vi "Report.FileName.vi"(8 "error in (no error)":errorcluster caption="错误输入（无错误）", 11 "路径":path) -> (0 "error out":errorcluster caption="错误输出", 2 "处理文件数量":u32, 3 "ok?":bool)   [LabVIEW 2012, in "Lib_UEL.ATE.lvlib" / "Lib_Report.lvlib"]
uses:
  <vilib>/regexp/Match Regular Expression.xnode
  Lib_Report.lvlib
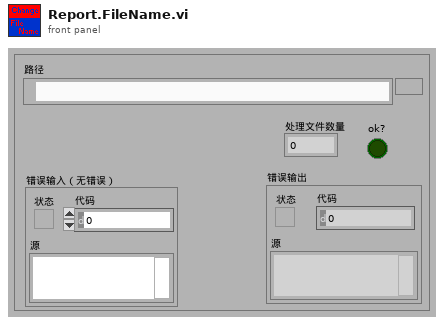
[diagram p1: front panel]
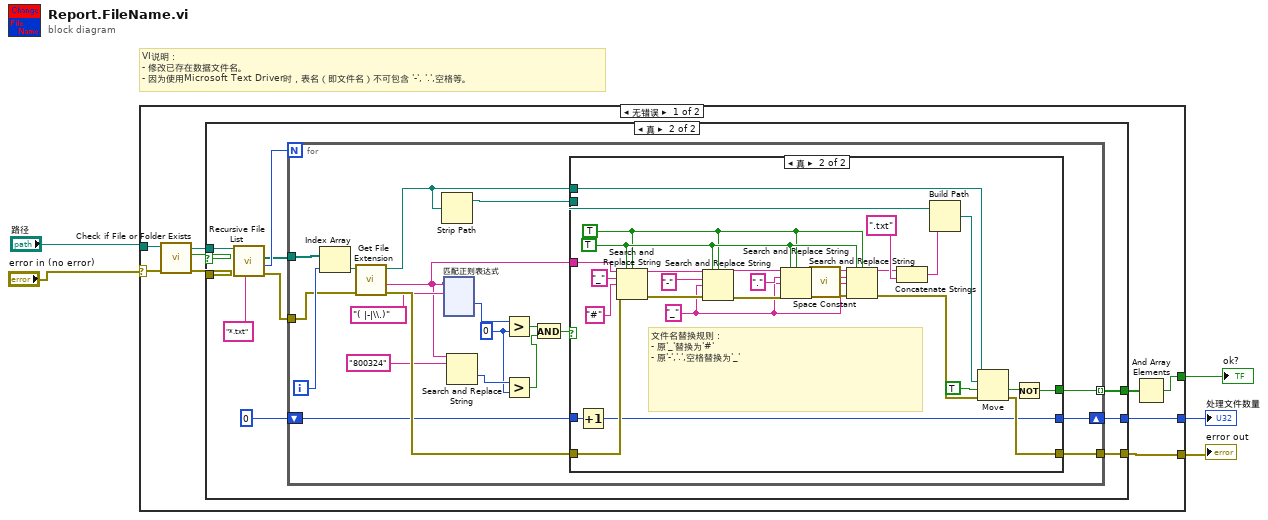
[diagram p0: block diagram]
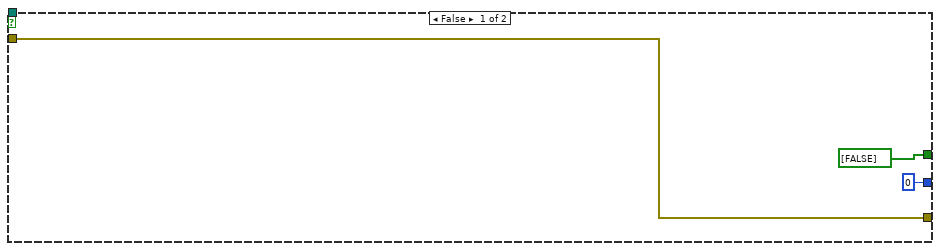
[diagram p2: hidden frame]
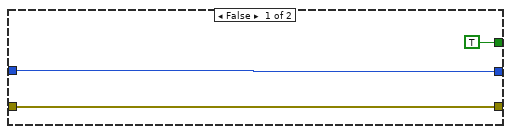
[diagram p3: hidden frame]
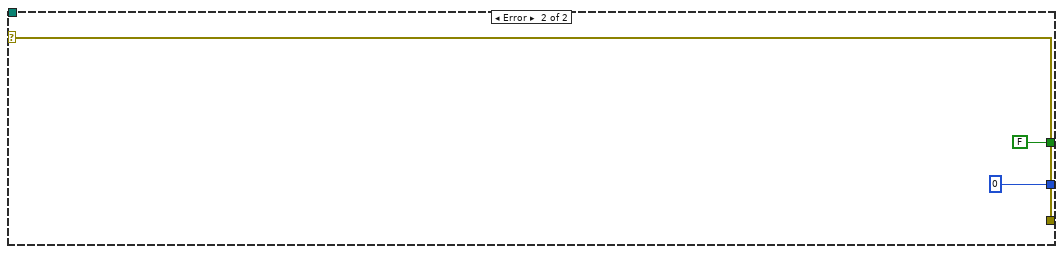
[diagram p4: hidden frame]
diagram:
  # "VI说明：\n- 修改已存在数据文件名。\n- 因为使用Microsoft Text Driver时，表名（即文件名）不可包含 '-', '.',空格等。"
  n1 = case shown="无错误" "error in (no error)" {
    selector: "error in (no error)" -> [w13 w193]
    tunnel: "路径" -> [w14 _]
    tunnel: [w9 w193] -> w3
    tunnel: [w8 u32 0 ("y")] -> w2
    tunnel: [w6 FALSE] -> w1
    frame No Error {
      n2 = call <vilib>:"Check if File or Folder Exists.vi"("error in (no error)"=w13, "path"=w14) -> ("error out"=w11:errorcluster, "file or folder exists?"=w12:bool, "dup path"=w10:path)  [unwired: 7 in]
      n3 = case shown="真" w12 {
        tunnel: w11 -> [w17 w27]
        tunnel: w10 -> [_ w22]
        tunnel: [w17 w21] -> w9
        tunnel: [u32 0 ("y") w19] -> w8
        tunnel: [bool[] [FALSE] w18] -> w7
        frame False {
        }
        frame True {
          n4 = call <vilib>:"Recursive File List.vi"("pattern"="*.txt", "error in (no error)"=w27, "Folder Path"=w22) -> ("error out"=w23:errorcluster, "Number of Files"=w25:i32, "All Files in Dir"=w24:path[])  [unwired: 4 in, 2 out]
          n5 = for {
            N: w25 -> [_]
            tunnel: w24 -> [w47]
            tunnel: w23 -> [w43]
            tunnel: [w45] -> w21
            shift-right: [w38] -> w19
            shift-left: u32 0 ("y") -> [w39]
            tunnel: [w37] -> w18 mode=indexing
            i -> [w46]
            w32 = 0 ("y")
            n6 = Index Array(array=w47, index=w46) -> (element=w44:path)
            n7 = call <vilib>:"Get File Extension.vi"("error in (no error)"=w43, "file"=w44) -> ("error out"=w40:errorcluster, "filename without extension"=w28:string, "dup file"=w42:path)  [unwired: 6 in, 1 out]
            n8 = Strip Path(path=w42) -> (stripped path=w41:path)  [unwired: 1 out]
            n9 = xnode "匹配正则表达式"("输入字符串"=w28, "正则表达式"="( |-|\\.)") -> ("匹配后偏移量"=w35:i32)  [unwired: 4 in, 4 out]
            n10 = Search and Replace String(input string=w28, search string="800324" ("搜索字符串")) -> (offset past replacement=w33:i32)  [unwired: 6 in, 3 out]
            n11 = Greater?(x=w35, y=w32) -> (0:w31:bool)
            n12 = Greater?(x=w33, y=w32) -> (0:w30:bool)
            n13 = And(x=w31, y=w30) -> (x .and. y?=w29:bool)
            n14 = case shown="真" w29 {
              tunnel: w28 -> [_ w188]
              tunnel: w41 -> [_ w181]
              tunnel: w42 -> [_ w165]
              tunnel: [w161 w180] -> w45
              tunnel: w40 -> [w161 w175]
              tunnel: w39 -> [w160 w167]
              tunnel: [w160 w166] -> w38
              tunnel: [TRUE ("cancelled") w163] -> w37
              frame False {
              }
              frame True {
                w162 = "_" ("搜索字符串")
                w170 = TRUE ("忽略大小写？(F)")
                w171 = TRUE ("替换全部？(F)")
                # "文件名替换规则：\n- 原'_'替换为'#'\n- 原'-','.',空格替换为'_'"
                n15 = Increment(x=w167) -> (x+1=w166:u32)
                n16 = Search and Replace String(replace all?=w171, case sensitive?=w170, input string=w188, search string="_" ("搜索字符串"), replace string="#" ("输入字符串"), error in=w175) -> (result string=w187:string, error out=w185:errorcluster)  [unwired: 2 in, 2 out]
                n17 = Search and Replace String(replace all?=w171, case sensitive?=w170, input string=w187, search string="-" ("搜索字符串"), replace string=w162, error in=w185) -> (result string=w183:string, error out=w184:errorcluster)  [unwired: 2 in, 2 out]
                n18 = Search and Replace String(replace all?=w171, case sensitive?=w170, input string=w183, search string="." ("搜索字符串"), replace string=w162, error in=w184) -> (result string=w169:string, error out=w174:errorcluster)  [unwired: 2 in, 2 out]
                n19 = call <vilib>:"Space Constant.vi"() -> ("String"=w168:string)
                n20 = Search and Replace String(replace all?=w171, case sensitive?=w170, input string=w169, search string=w168, replace string=w162, error in=w174) -> (result string=w172:string, error out=w173:errorcluster)  [unwired: 2 in, 2 out]
                n21 = Concatenate Strings(w172, ".txt" ("pattern")) -> (w176:string)
                n22 = Build Path(base path=w181, name or relative path=w176) -> (appended path=w179:path)
                n23 = Move(source path=w165, error in=w173, 9:TRUE ("覆盖(F)"), 10:w179) -> (error out=w180:errorcluster, 1:w164:bool)  [unwired: 1 in, 1 out]
                n24 = Not(x=w164) -> (.not. x?=w163:bool)
              }
            }
          }
        }
      }
      n25 = And Array Elements(Boolean array=w7) -> (logical AND=w6:bool)
    }
    frame Error {
    }
  }
  "error out" <- w3
  "处理文件数量" <- w2
  "ok?" <- w1
